vi "Embed Image.vi"(8 "error in (no error)":errorcluster, 10 "Pict Refnum":refnum<vi>, 11 "ImagePath":path) -> (0 "error out":errorcluster)   [LabVIEW 2023, in "EmbedImage.lvlib" / "EmbedImage.lvclass"]
doc: "This routine embeds image from the provided path to the provided reference"
uses:
  Library/EmbedImage.lvclass
  Library/EmbedImage.lvclass/EmbedImage.ctl
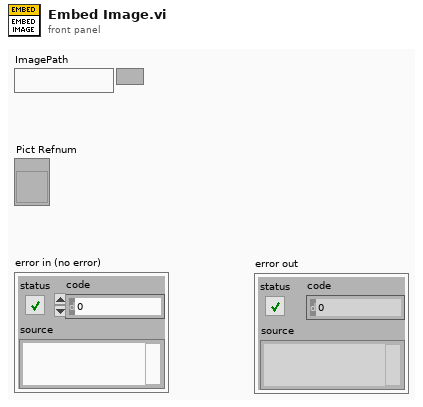
[diagram p1: front panel]
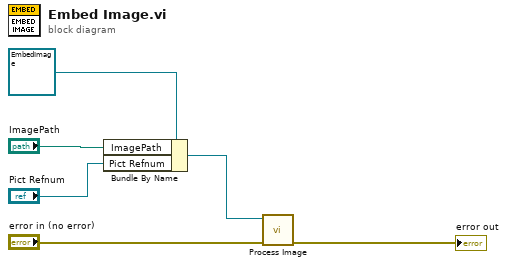
[diagram p0: block diagram]
diagram:
  n1 = Bundle By Name(cluster=refnum<class "EmbedImage.lvclass"> refnum ("EmbedImage.lvlib:EmbedImage.lvclass"), "ImagePath"="ImagePath", "Pict Refnum"="Pict Refnum") -> (w3:refnum<class "EmbedImage.lvclass">)
  n2 = call "Process Image.vi"("error in (no error)"="error in (no error)", "EmbedImage in"=w3) -> ("error out"=→"error out":errorcluster)  [unwired: 8 in, 1 out]
